vi "Set Path in Launcher.vi"(8 "error in":errorcluster, 11 "launcher path":path) -> (0 "error out":errorcluster)   [LabVIEW 2020]
doc: "Uses scripting to set the path the icon editor launcher should use to launch the source editor."
uses:
  <vilib>/Utility/traverseref.llb/TRef TravTarget.ctl
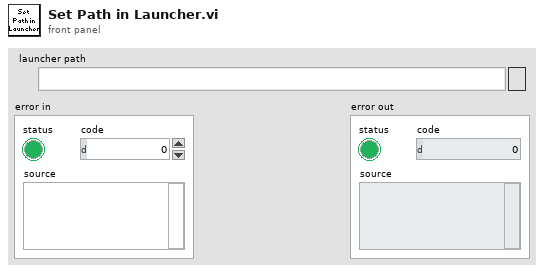
[diagram p1: front panel]
types:
  T1 = typedef "TRef TravTarget.ctl" = enum16{"FP", "BD", "Other"}
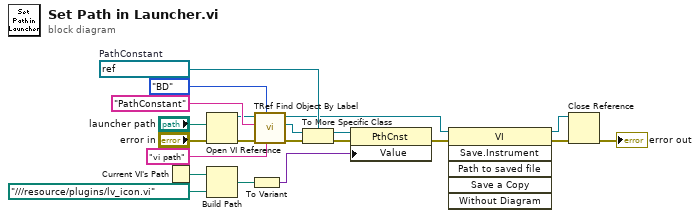
[diagram p0: block diagram]
diagram:
  w7 = refnum<vi> refnum  # PathConstant
  n1 = Current VI's Path() -> (path=w3:path)
  n2 = Open VI Reference(vi path="launcher path", error in (no error)="error in") -> (vi reference=w9:refnum<vi>, error out=w20:errorcluster)  [unwired: 4 in]
  n3 = Build Path(base path=w3, name or relative path=path "../../../resource/plugins/lv_icon.vi") -> (appended path=w1:path)
  n4 = To Variant(anything=w1) -> (Variant=w6:variant)
  n5 = call <vilib>:"TRef Find Object By Label.vi"("Label"="vi path", "Traverse Target"=TRef_TravTarget."BD", "error in (no error)"=w20, "Class Name"="PathConstant", "VI Ref"=w9) -> ("error out"=w17:errorcluster, "Found Obj Ref"=w10:refnum<vi>, "dup VI Ref"=w5:refnum<vi>)  [unwired: 3 in, 1 out]
  n6 = To More Specific Class(target class=w7, reference=w10, error in=w17) -> (specific class reference=w8:refnum<vi>, error out=w16:errorcluster)
  n7 = property class="PthCnst"(reference=w8, error in=w16, "Value"=w6) -> (error out=w19:errorcluster)  [unwired: 1 out]
  n8 = invoke class="VI" method="Save.Instrument"(reference=w5, error in=w19) -> (reference out=w4:refnum<vi>, error out=w15:errorcluster)  [unwired: 4 in, 4 out]
  n9 = Close Reference(reference=w4, error in (no error)=w15) -> (error out=→"error out":errorcluster)
